vi "StateAlarmManagement.vi"(0 "Master State In":T1(ring)) -> ()   [LabVIEW 2023]
doc: "This VI manages the Master ALARM and master CAUTION states for the robot."
uses:
  GlobalMiscellaneous.vi
  GlobalPoseAndTargeting.vi
  GlobalDriverStationData.vi
  GlobalAutonomous.vi
  GlobalDrivebase.vi
  GlobalElevator.vi
  GlobalShooter.vi
  GlobalNoteHandling.vi
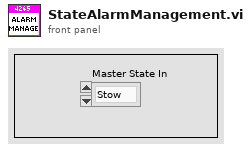
[diagram p1: front panel]
types:
  T1 = enum16{"Stow", "Speaker", "Amp", "Climbing", "Trap"}
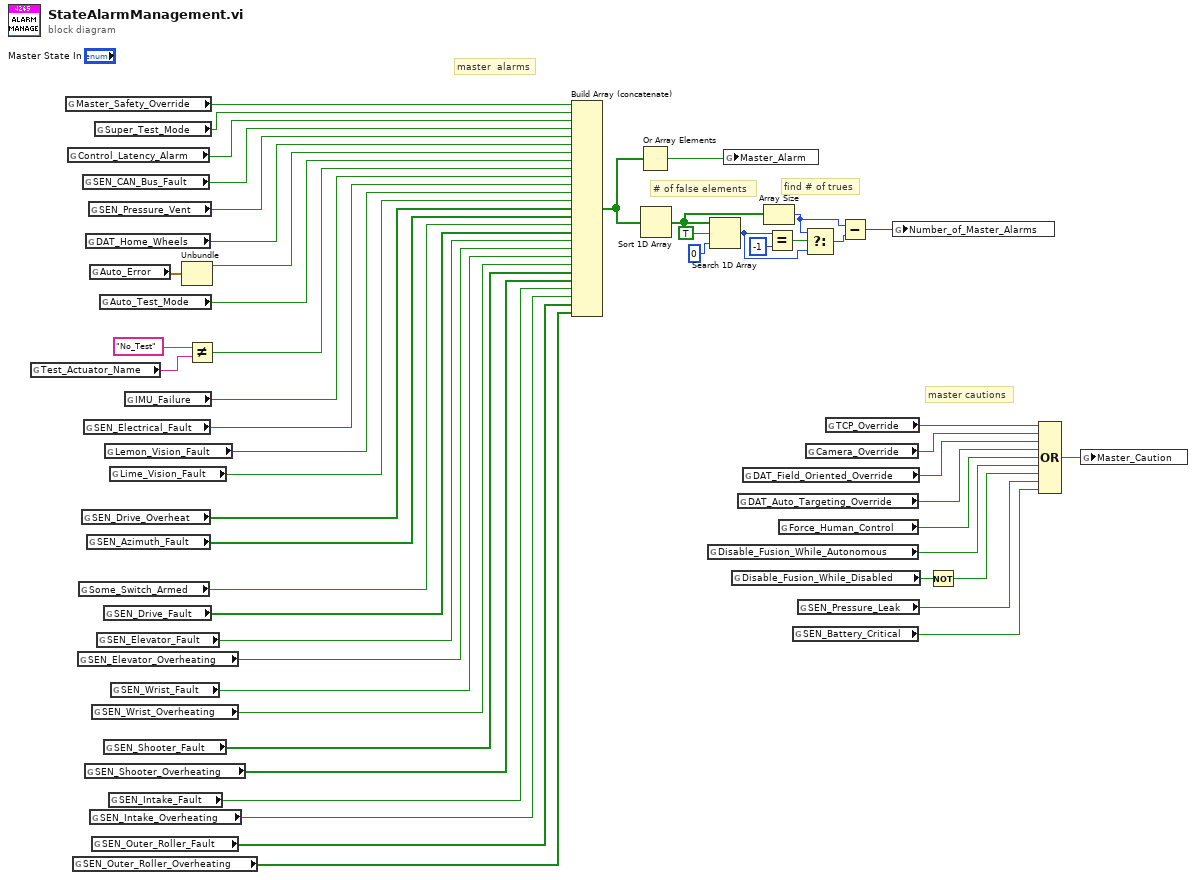
[diagram p0: block diagram]
diagram:
  # "master cautions"
  # "master  alarms"
  # "# of false elements"
  # "find # of trues"
  n1 = global read "GlobalDriverStationData.vi" "Test_Actuator_Name"() -> (w46:string)
  n2 = global read "GlobalDriverStationData.vi" "Master_Safety_Override"() -> (w52:bool)
  n3 = global read "GlobalMiscellaneous.vi" "Control_Latency_Alarm"() -> (w27:bool)
  n4 = global read "GlobalNoteHandling.vi" "SEN_Outer_Roller_Overheating"() -> (w1:bool[])
  n5 = global read "GlobalElevator.vi" "SEN_Elevator_Overheating"() -> (w9:bool)
  n6 = global read "GlobalDriverStationData.vi" "Some_Switch_Armed"() -> (w22:bool)
  n7 = global read "GlobalDrivebase.vi" "SEN_Drive_Overheat"() -> (w24:bool[])
  n8 = global read "GlobalMiscellaneous.vi" "SEN_CAN_Bus_Fault"() -> (w26:bool)
  n9 = global read "GlobalMiscellaneous.vi" "SEN_Electrical_Fault"() -> (w28:bool)
  n10 = global read "GlobalShooter.vi" "SEN_Shooter_Overheating"() -> (w5:bool[])
  n11 = global read "GlobalDrivebase.vi" "DAT_Home_Wheels"() -> (w29:bool)
  n12 = global read "GlobalDrivebase.vi" "SEN_Azimuth_Fault"() -> (w23:bool[])
  n13 = global read "GlobalMiscellaneous.vi" "SEN_Pressure_Vent"() -> (w25:bool)
  n14 = global read "GlobalAutonomous.vi" "Auto_Error"() -> (w50:errorcluster)
  n15 = global read "GlobalNoteHandling.vi" "SEN_Intake_Overheating"() -> (w3:bool)
  n16 = global read "GlobalShooter.vi" "SEN_Wrist_Overheating"() -> (w6:bool)
  n17 = global read "GlobalNoteHandling.vi" "SEN_Outer_Roller_Fault"() -> (w2:bool[])
  n18 = global read "GlobalDriverStationData.vi" "Super_Test_Mode"() -> (w51:bool)
  n19 = global read "GlobalElevator.vi" "SEN_Elevator_Fault"() -> (w10:bool)
  n20 = global read "GlobalDriverStationData.vi" "Auto_Test_Mode"() -> (w48:bool)
  n21 = global read "GlobalDrivebase.vi" "SEN_Drive_Fault"() -> (w12:bool[])
  n22 = global read "GlobalShooter.vi" "SEN_Shooter_Fault"() -> (w7:bool[])
  n23 = global read "GlobalPoseAndTargeting.vi" "Lemon_Vision_Fault"() -> (w43:bool)
  n24 = global read "GlobalNoteHandling.vi" "SEN_Intake_Fault"() -> (w4:bool)
  n25 = global read "GlobalPoseAndTargeting.vi" "Lime_Vision_Fault"() -> (w11:bool)
  n26 = global read "GlobalShooter.vi" "SEN_Wrist_Fault"() -> (w8:bool)
  n27 = global read "GlobalPoseAndTargeting.vi" "IMU_Failure"() -> (w44:bool)
  n28 = Unbundle(w50) -> ("status"=w49:bool)  [unwired: 2 out]
  n29 = Not Equal?(x="No_Test", y=w46) -> (x != y?=w45:bool)
  n30 = Build Array (concatenate)(w52, w51, w27, w26, w25, w29, w49, w48, w45, w44, w28, w43, w11, w24, w23, w22, w12, w10, w9, w8, w6, w7, w5, w4, w3, w2, w1) -> (w34:bool[])
  n31 = Or Array Elements(Boolean array=w34) -> (logical OR=w33:bool)
  n32 = Sort 1D Array(array=w34) -> (sorted array=w39:bool[])
  n33 = global read "GlobalDriverStationData.vi" "Disable_Fusion_While_Autonomous"() -> (w17:bool)
  n34 = Search 1D Array(1D array=w39, element=TRUE, start index (0)=0) -> (index of element=w42:i32)
  n35 = global write "GlobalMiscellaneous.vi" "Master_Alarm"(w33) -> ()
  n36 = global read "GlobalDriverStationData.vi" "Disable_Fusion_While_Disabled"() -> (w16:bool)
  n37 = global read "GlobalDrivebase.vi" "DAT_Auto_Targeting_Override"() -> (w19:bool)
  n38 = global read "GlobalDrivebase.vi" "DAT_Field_Oriented_Override"() -> (w20:bool)
  n39 = Array Size(array=w39) -> (size(s)=w41:i32)
  n40 = Equal?(x=w42, y=-1) -> (x = y?=w38:bool)
  n41 = global read "GlobalDriverStationData.vi" "Force_Human_Control"() -> (w18:bool)
  n42 = global read "GlobalMiscellaneous.vi" "SEN_Battery_Critical"() -> (w13:bool)
  n43 = global read "GlobalMiscellaneous.vi" "SEN_Pressure_Leak"() -> (w14:bool)
  n44 = Select(t=w41, s=w38, f=w42) -> (s? t:f=w40:i32)
  n45 = global read "GlobalDriverStationData.vi" "Camera_Override"() -> (w21:bool)
  n46 = global read "GlobalDriverStationData.vi" "TCP_Override"() -> (w31:bool)
  n47 = Subtract(x=w41, y=w40) -> (x-y=w32:i32)
  n48 = global write "GlobalMiscellaneous.vi" "Number_of_Master_Alarms"(w32) -> ()
  n49 = Not(x=w16) -> (.not. x?=w15:bool)
  n50 = Compound Arithmetic op=OR(w31, w21, w20, w19, w18, w17, w15, w14, w13) -> (w30:bool)
  n51 = global write "GlobalMiscellaneous.vi" "Master_Caution"(w30) -> ()
